vi "setup experiment.vi"(8 "error in (no error)":errorcluster, 11 "Cascade in":refnum<class "Cascade.lvclass">) -> (0 "error out":errorcluster, 3 "Cascade out":refnum<class "Cascade.lvclass">)   [LabVIEW 2012, in "Cascade.lvclass"]
uses:
  Cascade.lvclass
  Cascade.lvclass/Cascade.ctl
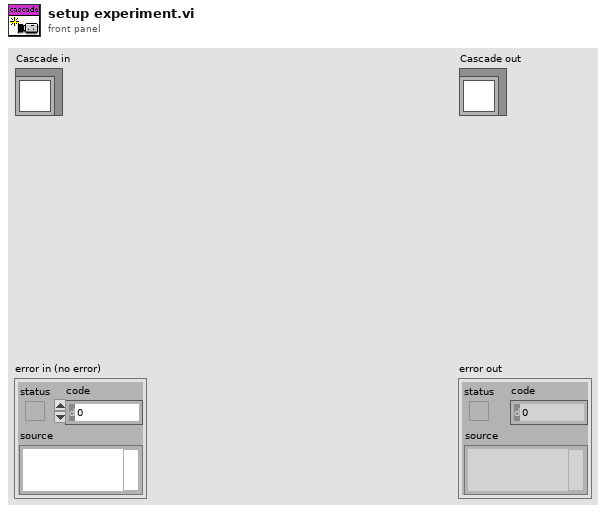
[diagram p1: front panel]
types:
  T1 = typedef "Cascade.lvclass/acquire flag.ctl" = u32
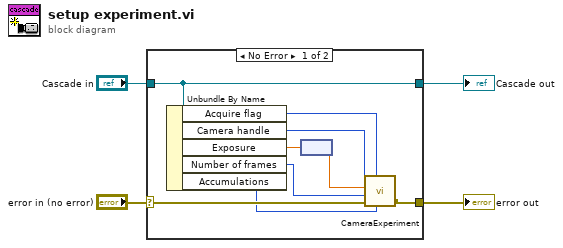
[diagram p0: block diagram]
diagram:
  n1 = case shown="No Error" "error in (no error)" {
    selector: "error in (no error)" -> [w13 w15]
    tunnel: [w5 w15] -> w3
    tunnel: [w12 w14] -> w1
    tunnel: "Cascade in" -> [w12 w14]
    frame No Error {
      n2 = Unbundle By Name(w12) -> ("Acquire flag"=w7:T1, "Camera handle"=w11:u32, "Exposure"=w10:dbl[unit], "Number of frames"=w8:u32, "Accumulations"=w6:u32)
      n3 = node(w10) -> (w9:dbl)
      n4 = call <userlib>:"CameraExperiment.vi"("Number of Accumulations"=w6, "Acquire / Focus Flag"=w7, "error in"=w13, "Number of Images"=w8, "Exposure (sec)"=w9, "Camera Handle"=w11) -> ("error out"=w5:errorcluster)  [unwired: 1 out]
    }
    frame Error {
    }
  }
  "error out" <- w3
  "Cascade out" <- w1
